vi "Destroy.vi"(8 "Error In":errorcluster, 11 "reference in":refnum<class "Electronic Datasheet.lvclass">) -> (0 "Error Out":errorcluster, 3 "reference out":refnum<class "Electronic Datasheet.lvclass">)   [LabVIEW 2019, in "Electronic Datasheet.lvlib" / "Electronic Datasheet.lvclass"]
uses:
  Electronic Datasheet.lvclass
  Core/Sorted Object Dictionary/Sorted Object Dictionary.lvclass
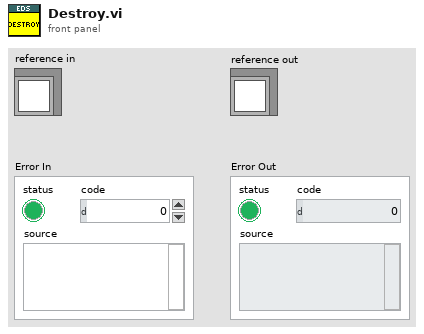
[diagram p1: front panel]
types:
  T1 = typedef "Electronic Datasheet.lvlib/Electronic Datasheet.lvclass/ObjectAttributes.ctl" = cluster{"EDS File Path":path, "Object Dict":refnum<class "Dictionary.lvclass">, "Sorted Object Dict":refnum<class "Sorted Object Dictionary.lvclass">, "Device Info":refnum<class "Device Info.lvclass">, "File Info":refnum<class "File Info.lvclass">}
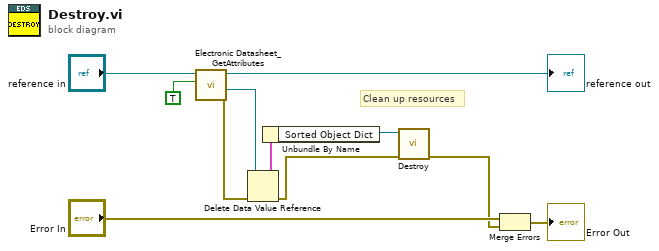
[diagram p0: block diagram]
diagram:
  # "Clean up resources"
  n1 = call "Electronic Datasheet_GetAttributes.vi"("OnlyGetDvrReference(False)"=TRUE, "reference in"="reference in") -> ("Error Out"=w8:errorcluster, "DataRef"=w7:refnum<data-value>, "reference out"=→"reference out":refnum<class "Electronic Datasheet.lvclass">)  [unwired: 6 in, 1 out]
  n2 = Delete Data Value Reference(data value reference=w7, error in=w8) -> (data value=w4:T1, error out=w2:errorcluster)
  n3 = Unbundle By Name(w4) -> ("Sorted Object Dict"=w3:refnum<class "Sorted Object Dictionary.lvclass">)
  n4 = call "Destroy.vi"("error in"=w2, "Sorted Object Dictionary in"=w3) -> ("error out"=w1:errorcluster)  [unwired: 8 in, 1 out]
  n5 = Merge Errors("Error In", w1) -> (→"Error Out":errorcluster)
